vi "Append Dictionary Element.vi"(8 "error in (no error)":errorcluster, 9 "value":variant, 10 "key":string, 11 "Control Experiment in":refnum<class "Control Experiment.lvclass">) -> (0 "error out":errorcluster, 3 "Control Experiment out":refnum<class "Control Experiment.lvclass">)   [LabVIEW 2019, in "Control Experiment.lvclass"]
uses:
  Control Experiment.lvclass
  <userlib>/LevyLab/LV-Data/LV-Data/Typedefs/Dictionary--cluster.ctl
  Control Experiment.lvclass/Control Experiment.ctl
  <userlib>/_OpenG.lib/dictionary/dictionary.llb/Dictionary Update (by scalar value)__ogtk.vi
  <userlib>/LevyLab/LV-Data/LV-Data/LV-Data.lvclass
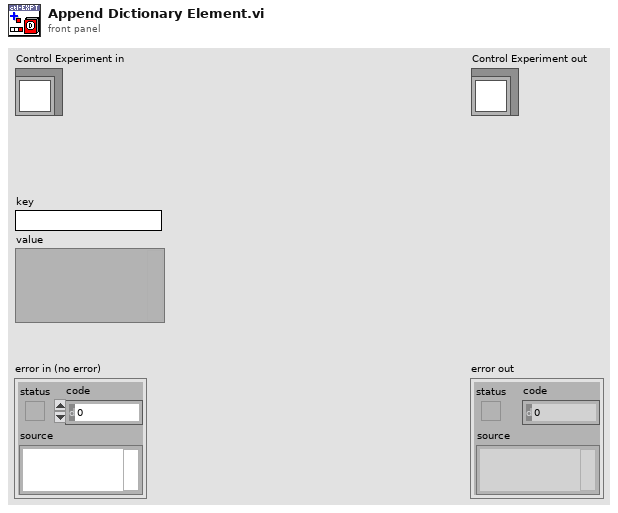
[diagram p1: front panel]
types:
  T1 = typedef "LV-Data.lvclass/Dictionary--cluster.ctl" = cluster{"key":string, "value":variant}
  T2 = typedef "Dictionary Object RefNum__ogtk.ctl" = refnum<k1>
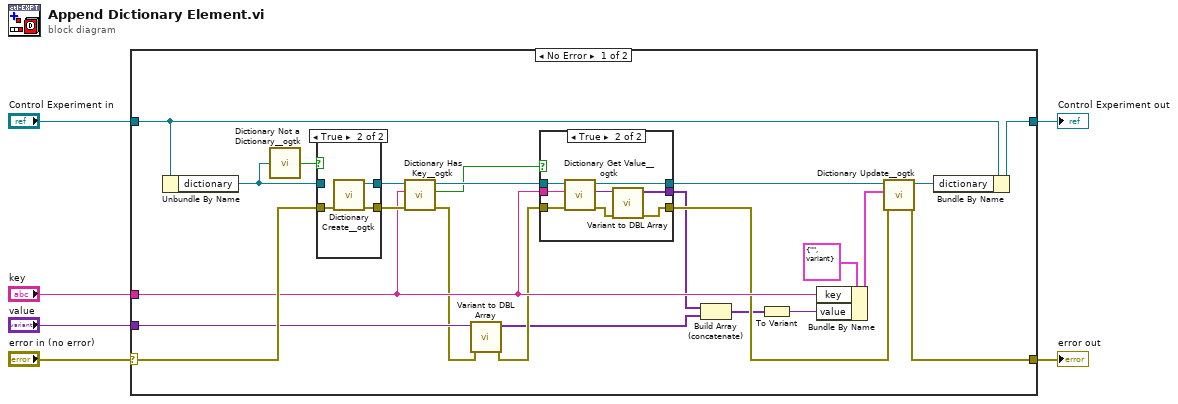
[diagram p0: block diagram]
diagram:
  n1 = case shown="No Error" "error in (no error)" {
    selector: "error in (no error)" -> [w25 w45]
    tunnel: [w27 w45] -> w5
    tunnel: [w29 w46] -> w3
    tunnel: "Control Experiment in" -> [w28 w46]
    tunnel: "key" -> [w19 _]
    tunnel: "value" -> [w15 _]
    frame No Error {
      n2 = Unbundle By Name(w28) -> ("dictionary"=w24:T2)
      n3 = call <userlib>:"Dictionary Not a Dictionary__ogtk.vi"("dictionary"=w24) -> ("not a dictionary?"=w26:bool)
      n4 = case shown="True" w26 {
        tunnel: [w31 w34] -> w23
        tunnel: w24 -> [w31 _]
        tunnel: [w30 w33] -> w22
        tunnel: w25 -> [w30 w32]
        frame False {
        }
        frame True {
          n5 = call <userlib>:"Dictionary Create__ogtk.vi"("error in (no error)"=w32) -> ("error out"=w33:errorcluster, "dictionary out"=w34:T2)  [unwired: 9 in]
        }
      }
      n6 = call <userlib>:"Dictionary Has Key__ogtk.vi"("error in (no error)"=w22, "key"=w19, "dictionary"=w23) -> ("error out"=w14:errorcluster, "Has Key?"=w18:bool, "dictionary out"=w21:T2)  [unwired: 6 in]
      n7 = call "Variant to DBL Array.vi"("error in (no error)"=w14, "value"=w15) -> ("error out"=w13:errorcluster, "Variant (1D array)"=w12:variant[])  [unwired: 8 in]
      n8 = case shown="True" w18 {
        tunnel: w21 -> [w35 w44]
        tunnel: w13 -> [w36 w43]
        tunnel: w19 -> [_ w42]
        tunnel: [w36 w38] -> w17
        tunnel: [w35 w41] -> w16
        tunnel: [_ w37] -> w11
        frame False {
        }
        frame True {
          n9 = call <userlib>:"Dictionary Get Value__ogtk.vi"("error in"=w43, "key"=w42, "dictionary"=w44) -> ("error out"=w39:errorcluster, "value"=w40:variant, "dictionary out"=w41:T2)  [unwired: 5 in, 1 out]
          n10 = call "Variant to DBL Array.vi"("error in (no error)"=w39, "value"=w40) -> ("error out"=w38:errorcluster, "Variant (1D array)"=w37:variant[])  [unwired: 8 in]
        }
      }
      n11 = Build Array (concatenate)(w11, w12) -> (w10:variant[])
      n12 = To Variant(anything=w10) -> (Variant=w20:variant)
      n13 = Bundle By Name(cluster=T1 {"key"="", "value"=variant} ("key-value"), "key"=w19, "value"=w20) -> (w7:T1)
      n14 = call-poly <userlib>:"Dictionary Update__ogtk.vi"("error in (no error)"=w17, "key-value"=w7, "dictionary"=w16) -> ("error out"=w27:errorcluster, "dictionary out"=w8:T2)  [unwired: 6 in, 1 out]
      n15 = Bundle By Name(cluster=w28, "dictionary"=w8) -> (w29:refnum<class "Control Experiment.lvclass">)
    }
    frame Error {
    }
  }
  "error out" <- w5
  "Control Experiment out" <- w3
